vi "Lectura de Voltaje con Arduino.vi"() -> ()   [LabVIEW 2014]
uses:
  <vilib>/LabVIEW Interface for Arduino/LabVIEW Interface for Arduino.lvlib
panel:
  in  "VISA resource name":refnum<visa-resource-name>
  in  "Horizontal Pointer Slide":u32(slide) scale=0.0..100.0
  out "Waveform Chart":dbl(graph)
  # "Adquisistion Time"
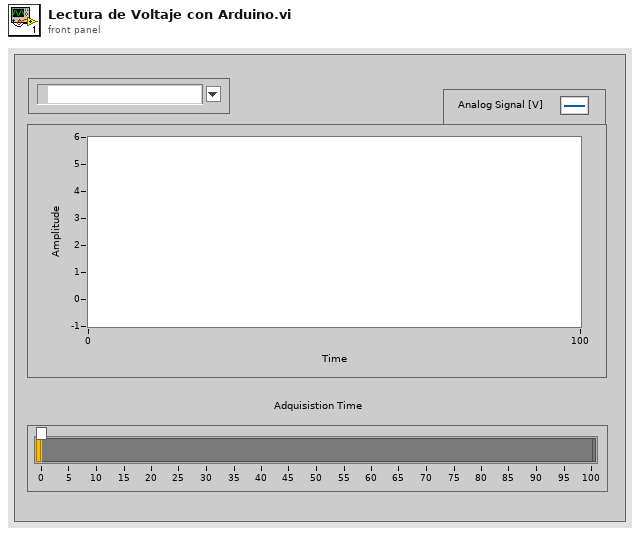
[diagram p1: front panel]
types:
  T1 = typedef "LabVIEW Interface for Arduino.lvlib/Arduino Resource.ctl" = cluster{"VISA resource":refnum<visa-resource-name>, "Board Type":T2, "Connection Type":enum8{"USB / Serial"}, "Bytes Per Packet (15)":u8}
  T2 = typedef "LabVIEW Interface for Arduino.lvlib/Board Type.ctl" = enum16{"Uno", "Dimuelanove w/Atmega 328", "Mega 2560"}
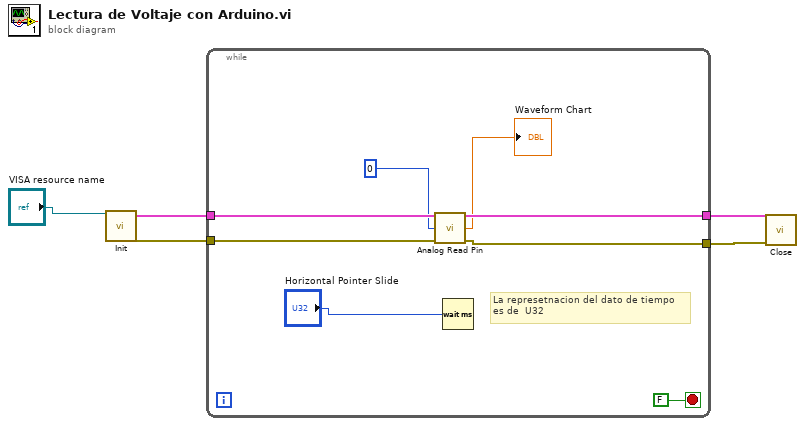
[diagram p0: block diagram]
diagram:
  n1 = call <vilib>:"Init.vi"("VISA resource"="VISA resource name") -> ("Arduino Resource"=w3:T1, "error out"=w5:errorcluster)  [unwired: 17 in]
  n2 = while {
    tunnel: w5 -> [w13]
    tunnel: [w12] -> w4
    tunnel: w3 -> [w11]
    tunnel: [w10] -> w2
    stop <- FALSE stop-if-true
    # "La represetnacion del dato de tiempo\nes de  U32"
    n3 = call <vilib>:"Analog Read Pin.vi"("Arduino Resource"=w11, "Analog Input Pin (0)"=u8 0, "error in"=w13) -> ("Arduino Resource"=w10:T1, "Voltage"=→"Waveform Chart":dbl, "error out"=w12:errorcluster)  [unwired: 10 in]
    n4 = Wait (ms)(milliseconds to wait="Horizontal Pointer Slide") -> ()  [unwired: 1 out]
  }
  n5 = call <vilib>:"Close.vi"("Arduino Resource"=w2, "error in"=w4) -> ()  [unwired: 13 in, 1 out]
